vi "init.vi"(8 "error in (no error)":errorcluster, 11 "Monochromator in":refnum<class "Monochromator.lvclass">) -> (0 "error out":errorcluster, 1 "Emulating":bool, 2 "Initialized":bool, 3 "Monochromator out":refnum<class "Monochromator.lvclass">, 4 "Status":string)   [LabVIEW 2016, in "Monochromator.lvclass"]
uses:
  Monochromator.lvclass
  Monochromator.lvclass/Monochromator.ctl
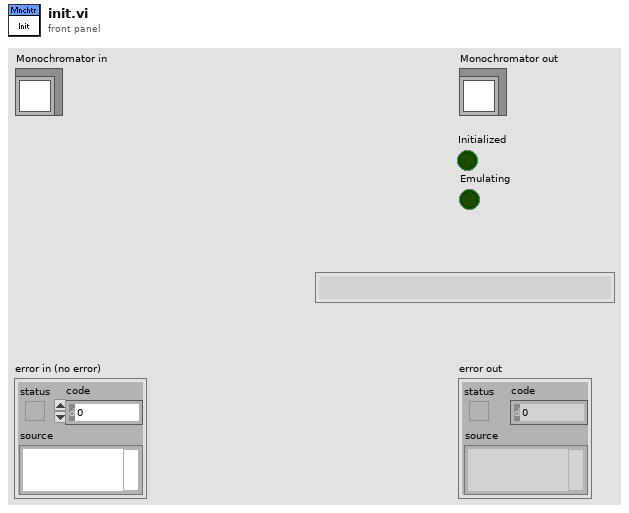
[diagram p1: front panel]
types:
  T1 = typedef "Settings.lvlib/ConfigurationTypedefs.lvlib/MonochromatorSettings.ctl" = cluster{"Force Init":bool, "WavelengthMin":T2, "WavelengthMax":T2, "SlitWidthMin":T3, "SlitWidthMax":T3, "timeout":dbl}
  T2 = typedef "wavelength.ctl" = dbl
  T3 = typedef "slitWidth.ctl" = dbl
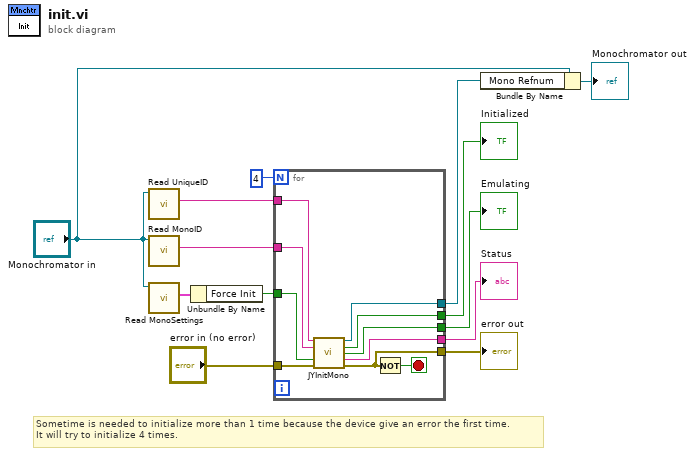
[diagram p0: block diagram]
diagram:
  # "Sometime is needed to initialize more than 1 time because the device give an error the first time.\nIt will try to initialize 4 times."
  n1 = call "Read UniqueID.vi"("Monochromator in"="Monochromator in") -> ("UniqueID"=w8:string)  [unwired: 8 in, 2 out]
  n2 = call "Read MonoID.vi"("Monochromator in"="Monochromator in") -> ("MonoID"=w5:string)  [unwired: 8 in, 2 out]
  n3 = call "Read MonoSettings.vi"("Monochromator in"="Monochromator in") -> ("Settings"=w3:T1)  [unwired: 8 in, 2 out]
  n4 = Unbundle By Name(w3) -> ("Force Init"=w2:bool)
  n5 = for {
    N: 4 -> [_]
    tunnel: [w22] -> w11
    tunnel: w8 -> [w19]
    tunnel: [w18] -> w7
    tunnel: "error in (no error)" -> [w23]
    tunnel: [w15] -> w12
    tunnel: w5 -> [w17]
    tunnel: [w20] -> w9
    tunnel: w2 -> [w16]
    tunnel: [w21] -> w10
    stop <- w14 stop-if-true
    n6 = call "JYInitMono.vi"("Unique ID"=w19, "Mono ID"=w17, "Force Init"=w16, "error in (no error)"=w23) -> ("Refnum out"=w18:refnum<k7>, "Initialized"=w22:bool, "Emulating"=w21:bool, "Status"=w20:string, "error out"=w15:errorcluster)  [unwired: 7 in]
    n7 = Not(x=w15) -> (.not. x?=w14:bool)
  }
  "error out" <- w12
  "Initialized" <- w11
  "Emulating" <- w10
  "Status" <- w9
  n8 = Bundle By Name(cluster="Monochromator in", "Mono Refnum"=w7) -> (→"Monochromator out":refnum<class "Monochromator.lvclass">)
